vi "FGV Stoermeldungen.vi"(6 "Aktion":T2, 8 "eintragen":bool, 9 "Zeitstempel":timestamp, 11 "Meldungs-Nummer":i32) -> (0 "Anzeige Array":T1[](array[typedef]), 1 "Queue-Inhalt":T1[](array[typedef]), 3 "Störmelde-Änderung":bool, 4 "Loggen in Datei":T1[](array[typedef]))   [LabVIEW 2020, in "Stoerungen.lvlib"]
uses:
  Stoerungen.lvlib
  FGV Stoermeldungen Aktion.ctl
  Stoermeldung.ctl
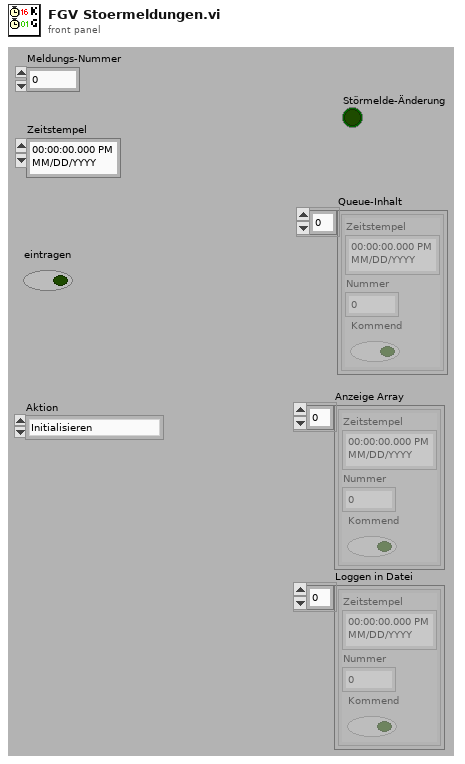
[diagram p1: front panel]
types:
  T1 = typedef "Stoerungen.lvlib/Stoermeldung.ctl" = cluster{"Zeitstempel":timestamp, "Nummer":i32, "Kommend":bool}
  T2 = typedef "Stoerungen.lvlib/FGV Stoermeldungen Aktion.ctl" = enum16{"Initialisieren", "kommend", "gehend", "lesen", "Queue leeren", "Queue freigeben", "in Datei loggen", "Änderung zurücksetzen"}
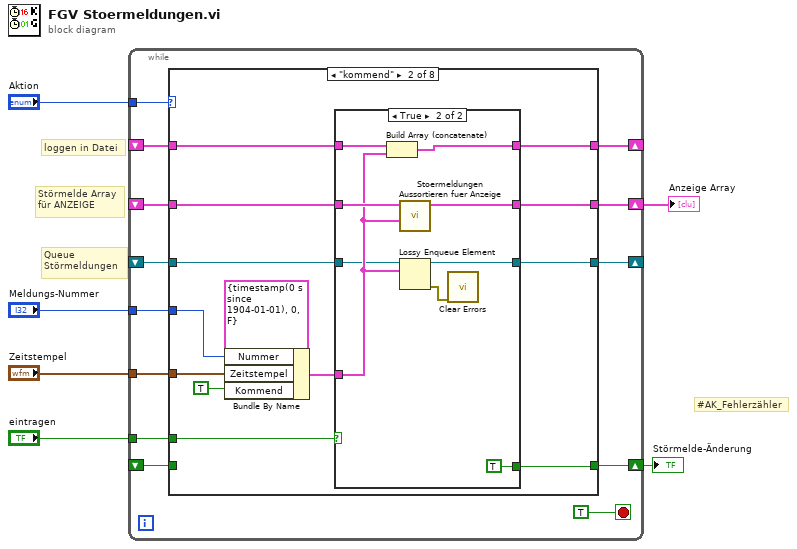
[diagram p0: block diagram]
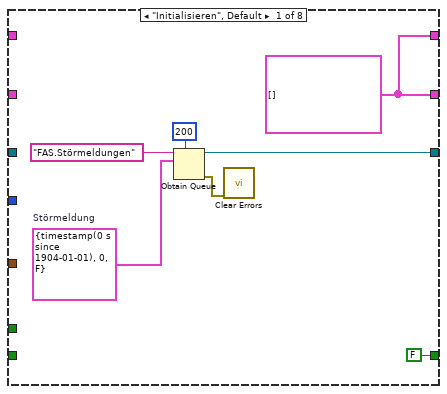
[diagram p2: hidden frame]
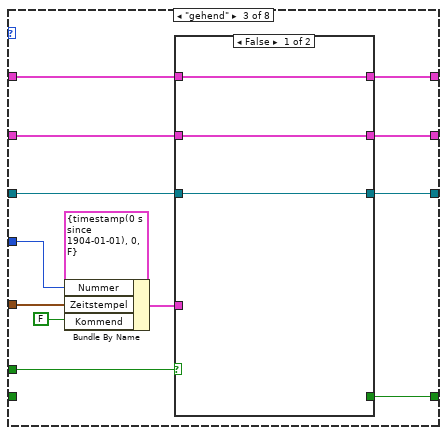
[diagram p4: hidden frame]
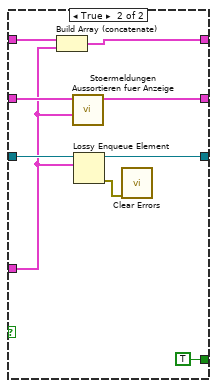
[diagram p5: hidden frame]
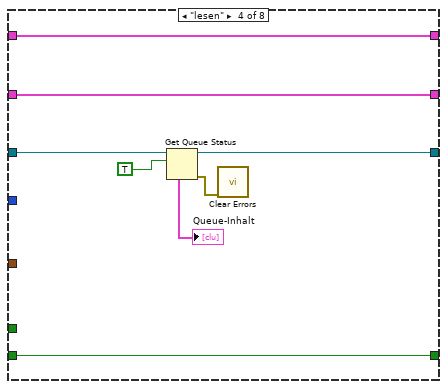
[diagram p6: hidden frame]
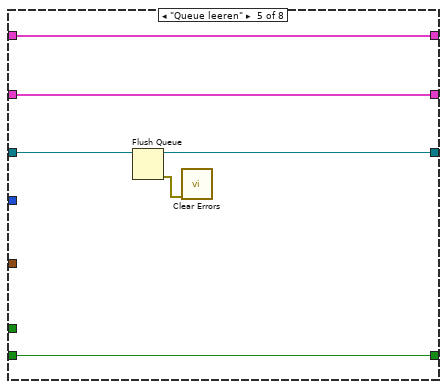
[diagram p7: hidden frame]
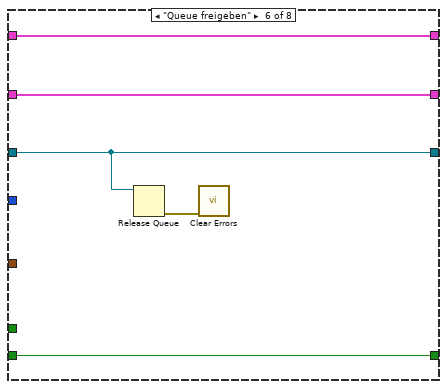
[diagram p8: hidden frame]
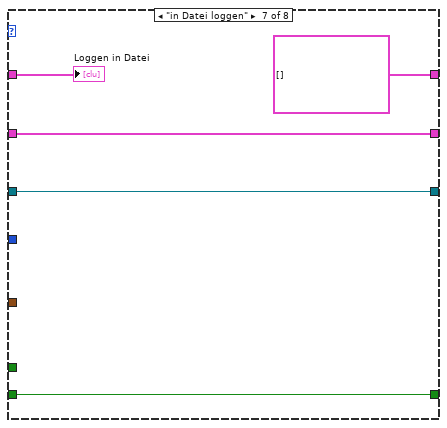
[diagram p9: hidden frame]
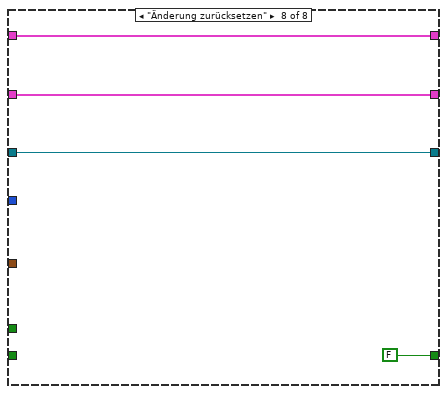
[diagram p10: hidden frame]
diagram:
  # "#AK_Fehlerzähler"
  # "loggen in Datei"
  # "Störmelde Array\nfür ANZEIGE"
  # "Queue\nStörmeldungen"
  n1 = while {
    tunnel: "Aktion" -> [w18]
    shift-right: [w17] -> _
    shift-left: _ -> [w16]
    tunnel: "Meldungs-Nummer" -> [w14]
    tunnel: "eintragen" -> [w13]
    tunnel: "Zeitstempel" -> [w15]
    shift-right: [w7] -> w2
    shift-left: _ -> [w12]
    shift-right: [w10] -> _
    shift-left: _ -> [w11]
    shift-right: [w8] -> w1
    shift-left: _ -> [w9]
    stop <- TRUE stop-if-true
    n2 = case shown="\"kommend\"" w18 {
      tunnel: [w25 w38 w63 w83 w89 w95 w99 w102] -> w17
      tunnel: w16 -> [_ w39 w64 w84 w90 w95 w99 w102]
      tunnel: w15 -> [_ w36 w61 _ _ _ _ _]
      tunnel: w14 -> [_ w35 w60 _ _ _ _ _]
      tunnel: w13 -> [_ w34 w59 _ _ _ _ _]
      tunnel: [w23 w30 w55 w80 w88 w94 w100 w103] -> w7
      tunnel: w12 -> [_ w31 w56 w80 w88 w94 w100 w103]
      tunnel: w11 -> [_ w29 w54 w79 w87 w93 w98 w104]
      tunnel: [w23 w28 w53 w79 w87 w93 T1[] [] ("Anzeige Array") w104] -> w10
      tunnel: w9 -> [_ _ _ w77 w85 w91 w96 _]
      tunnel: [FALSE w27 w52 w77 w85 w91 w96 FALSE] -> w8
      frame "Initialisieren", Default {
        w23 = T1[] [] ("Anzeige Array")
        w24 = T1 {"Zeitstempel"=timestamp(0 s since 1904-01-01), "Nummer"=0, "Kommend"=FALSE}  # Störmeldung
        n3 = Obtain Queue(max queue size (-1, unlimited)=200 ("Maximale Queue-Größe (-1, unbegrenzt)"), name (unnamed)="FAS.Störmeldungen" ("Name (unbenannt)"), element data type=w24) -> (queue out=w25:refnum<queue>, error out=w21:errorcluster)  [unwired: 2 in, 1 out]
        n4 = call <vilib>:"Clear Errors.vi"("error in (no error)"=w21) -> ()  [unwired: 5 in, 2 out]
      }
      frame "kommend" {
        n5 = Bundle By Name(cluster=T1 {"Zeitstempel"=timestamp(0 s since 1904-01-01), "Nummer"=0, "Kommend"=FALSE} ("Störmeldung"), "Nummer"=w35, "Zeitstempel"=w36, "Kommend"=TRUE) -> (w33:T1)
        n6 = case shown="True" w34 {
          tunnel: w39 -> [w42 w46]
          tunnel: [w42 w45] -> w38
          tunnel: w33 -> [_ w47]
          tunnel: w31 -> [w41 w51]
          tunnel: [w41 w50] -> w30
          tunnel: w29 -> [w40 w49]
          tunnel: [w40 w48] -> w28
          tunnel: [_ TRUE] -> w27
          frame False {
          }
          frame True {
            n7 = Build Array (concatenate)(w49, w47) -> (w48:T1[])
            n8 = call "Stoermeldungen Aussortieren fuer Anzeige.vi"("Störmeldung"=w47, "Anzeige Array"=w51) -> ("Anzeige Array"=w50:T1[])  [unwired: 9 in]
            n9 = Lossy Enqueue Element(queue=w46, element=w47) -> (queue out=w45:refnum<queue>, error out=w44:errorcluster)  [unwired: 1 in, 2 out]
            n10 = call <vilib>:"Clear Errors.vi"("error in (no error)"=w44) -> ()  [unwired: 5 in, 2 out]
          }
        }
      }
      frame "gehend" {
        n11 = Bundle By Name(cluster=T1 {"Zeitstempel"=timestamp(0 s since 1904-01-01), "Nummer"=0, "Kommend"=FALSE} ("Störmeldung"), "Nummer"=w60, "Zeitstempel"=w61, "Kommend"=FALSE) -> (w58:T1)
        n12 = case shown="False" w59 {
          tunnel: w64 -> [w67 w72]
          tunnel: [w67 w71] -> w63
          tunnel: w58 -> [_ w70]
          tunnel: w56 -> [w66 w76]
          tunnel: [w66 w75] -> w55
          tunnel: w54 -> [w65 w74]
          tunnel: [w65 w73] -> w53
          tunnel: [_ TRUE] -> w52
          frame False {
          }
          frame True {
            n13 = Build Array (concatenate)(w74, w70) -> (w73:T1[])
            n14 = call "Stoermeldungen Aussortieren fuer Anzeige.vi"("Störmeldung"=w70, "Anzeige Array"=w76) -> ("Anzeige Array"=w75:T1[])  [unwired: 9 in]
            n15 = Lossy Enqueue Element(queue=w72, element=w70) -> (queue out=w71:refnum<queue>, error out=w69:errorcluster)  [unwired: 1 in, 2 out]
            n16 = call <vilib>:"Clear Errors.vi"("error in (no error)"=w69) -> ()  [unwired: 5 in, 2 out]
          }
        }
      }
      frame "lesen" {
        n17 = Get Queue Status(queue=w84, return elements? (F)=TRUE ("Elemente ausgeben? (F)")) -> (queue out=w83:refnum<queue>, error out=w78:errorcluster, elements=→"Queue-Inhalt":T1[])  [unwired: 1 in, 5 out]
        n18 = call <vilib>:"Clear Errors.vi"("error in (no error)"=w78) -> ()  [unwired: 5 in, 2 out]
      }
      frame "Queue leeren" {
        n19 = Flush Queue(queue=w90) -> (queue out=w89:refnum<queue>, error out=w86:errorcluster)  [unwired: 1 in, 1 out]
        n20 = call <vilib>:"Clear Errors.vi"("error in (no error)"=w86) -> ()  [unwired: 5 in, 2 out]
      }
      frame "Queue freigeben" {
        n21 = Release Queue(queue=w95) -> (error out=w92:errorcluster)  [unwired: 1 in, 3 out]
        n22 = call <vilib>:"Clear Errors.vi"("error in (no error)"=w92) -> ()  [unwired: 5 in, 2 out]
      }
      frame "in Datei loggen" {
        "Loggen in Datei" <- w98
      }
      frame "Änderung zurücksetzen" {
      }
    }
  }
  "Anzeige Array" <- w2
  "Störmelde-Änderung" <- w1
